vi "Main.vi"() -> ()   [LabVIEW 2020]
doc: "This template is for the Queued Message Handler design pattern.\n\nThe Event Handling Loop generates messages based on user interface actions.\n\nThe Message Handling Loop processes messages generated by the Event Handling Loop, or by other messages. The messages are string values, so new messages can be added easily to the Message Cases case structure in the Message Handling Loop. Each message cluster can also provide an optional value for Message Data, which is a variant that can be converted to whatever message-specific data is required."
uses:
  controls/UI Data.ctl
  support/Message Queue/Message Cluster.ctl
  <extravilib>/ChannelInstances/Messenger-t'Message Queue.lvlib-Message Cluster.ctl'/Write With Abort.vi
  <extravilib>/ChannelInstances/Messenger-t'Message Queue.lvlib-Message Cluster.ctl'/Instantiate.vi
  <extravilib>/ChannelInstances/Messenger-t'Message Queue.lvlib-Message Cluster.ctl'/Endpoint.vi
  <extravilib>/ChannelInstances/Event Messenger-bool/Instantiate.vi
  <extravilib>/ChannelInstances/Event Messenger-bool/))Channel.vi
  <vilib>/Utility/error.llb/Error Cluster From Error Code.vi
  <vilib>/ErrorRing/Error Ring.xnode
  <extravilib>/ChannelInstances/Event Messenger-bool.lvlib
  support/Message Queue/Message Queue.lvlib
  <extravilib>/ChannelInstances/Messenger-t'Message Queue.lvlib-Message Cluster.ctl'.lvlib
panel:
  in  "Button sin":bool
  in  "Button ^":bool
  in  "Button )":bool
  in  "Button (":bool
  in  "Button Ans":bool
  in  "Button E":bool
  in  "Button /":bool
  in  "Button *":bool
  in  "Button const pi":bool
  in  "Button -":bool
  in  "Button const e":bool
  in  "Button +":bool
  in  "Button Clear":bool
  in  "Button Del":bool
  in  "Button =":bool
  in  "Button .":bool
  in  "Button 9":bool
  in  "Button 8":bool
  in  "Button 7":bool
  in  "Button 6":bool
  in  "Button 5":bool
  in  "Button 4":bool
  in  "Button 3":bool
  in  "Button 2":bool
  in  "Button 1":bool
  out "Display":string
  in  "Button 0":bool
  in  "Exit":bool
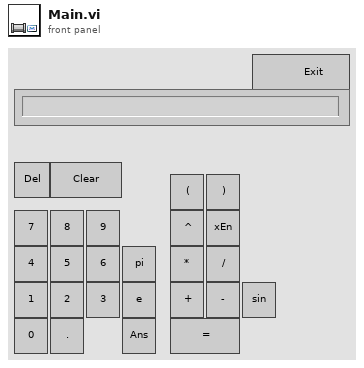
[diagram p1: front panel]
types:
  T1 = typedef "Message Queue.lvlib/Message Cluster.ctl" = cluster{"Message":string, "Message Data":variant}
  T2 = typedef "UI Data.ctl" = cluster{"Buttons to proces":string[], "Answer on display":bool, "Element type":string[], "Answer valid":bool, "Answer":string}
  T3 = typedef "Messenger-t'Message Queue.lvlib-Message Cluster.ctl'.lvlib/))Channel.ctl" = refnum<queue>
  T4 = cluster{"Strings to proces":string[], "Element type":string[]}
  T5 = cluster{"Buttons to proces":string[], "Element type":string[]}
  T6 = typedef "Event Messenger-bool.lvlib/))Channel.ctl" = refnum<queue>
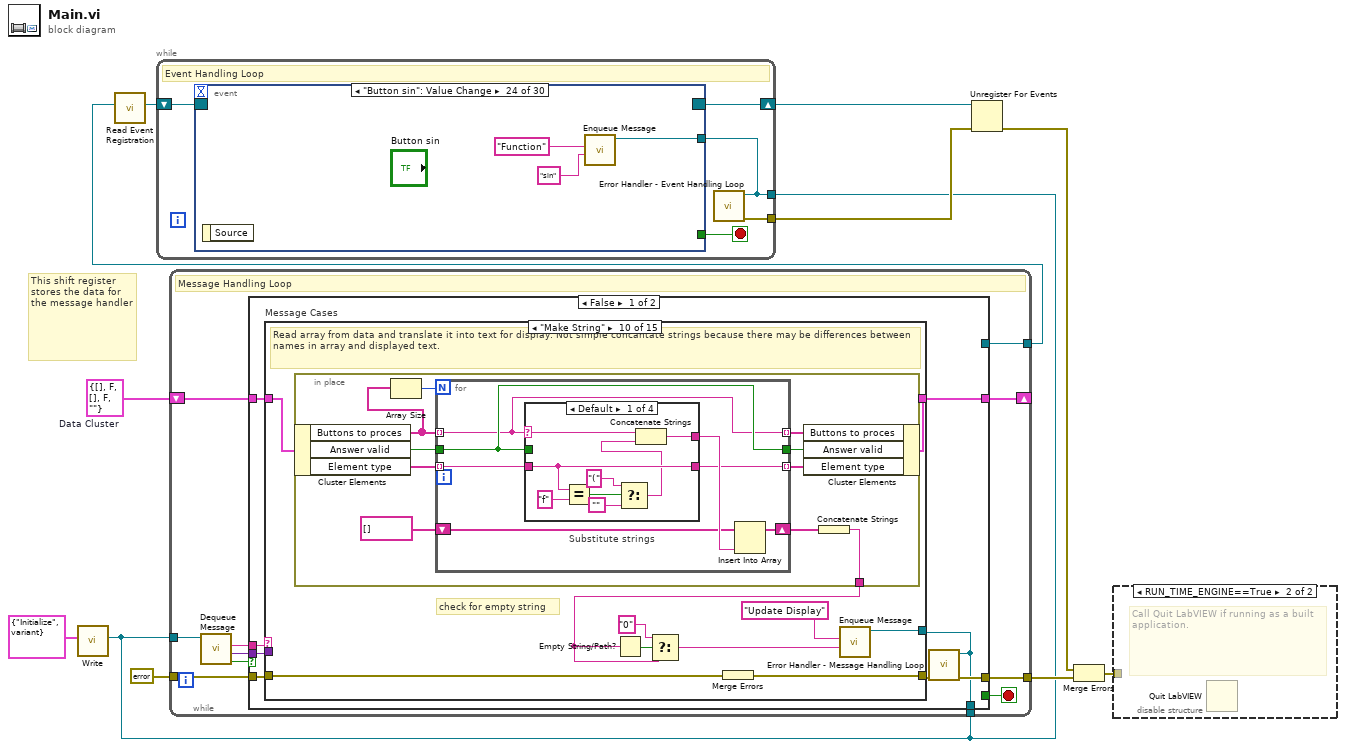
[diagram p0: block diagram]
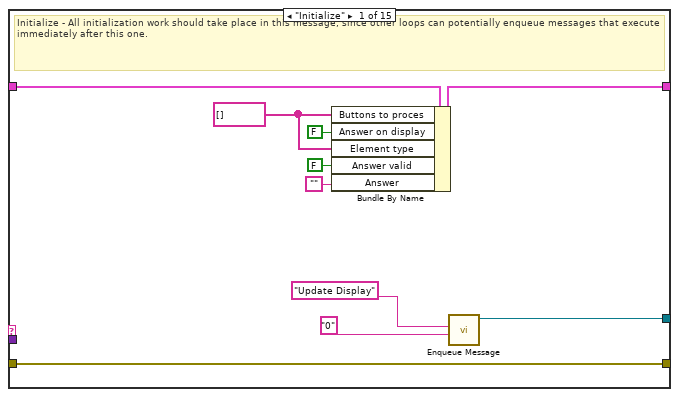
[diagram p2: hidden frame]
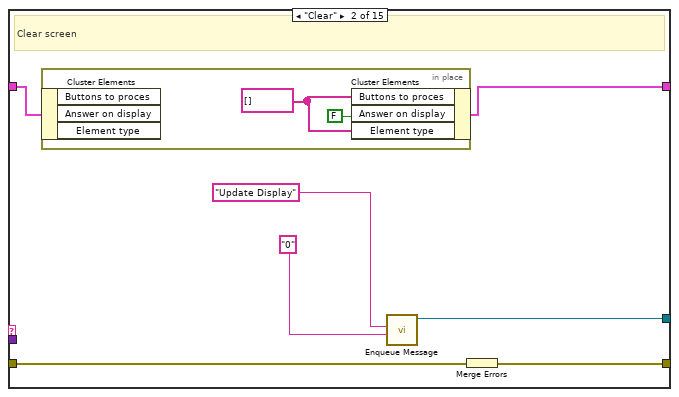
[diagram p3: hidden frame]
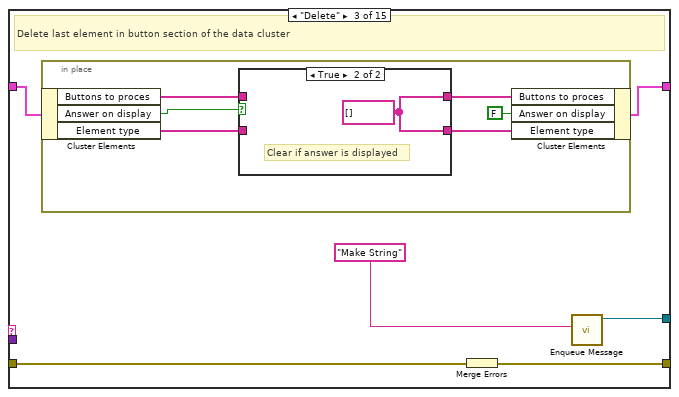
[diagram p4: hidden frame]
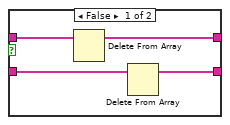
[diagram p5: hidden frame]
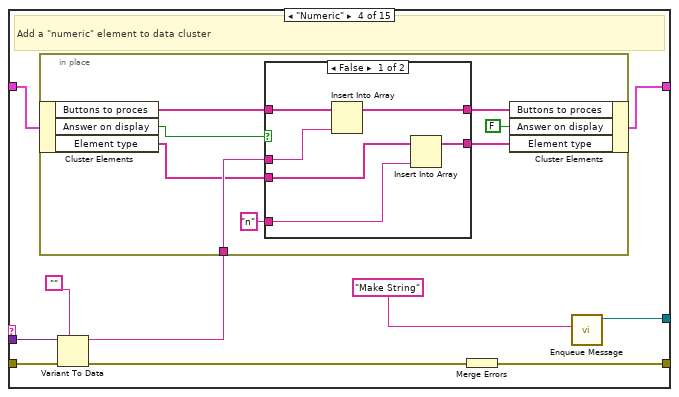
[diagram p6: hidden frame]
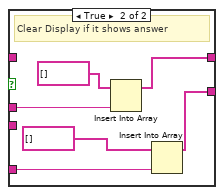
[diagram p7: hidden frame]
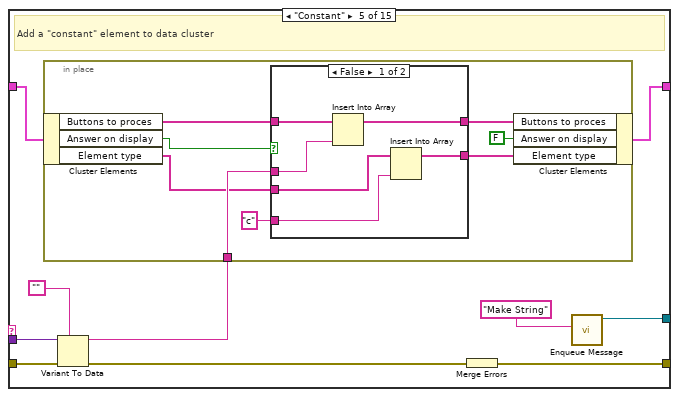
[diagram p8: hidden frame]
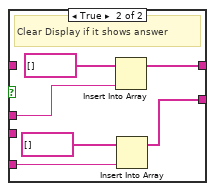
[diagram p9: hidden frame]
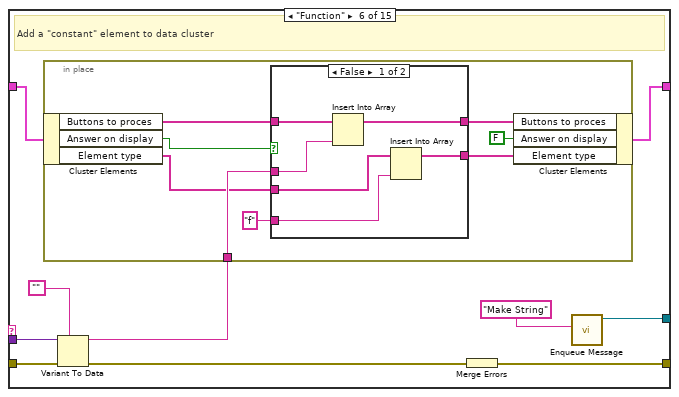
[diagram p10: hidden frame]
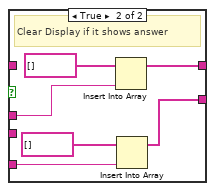
[diagram p11: hidden frame]
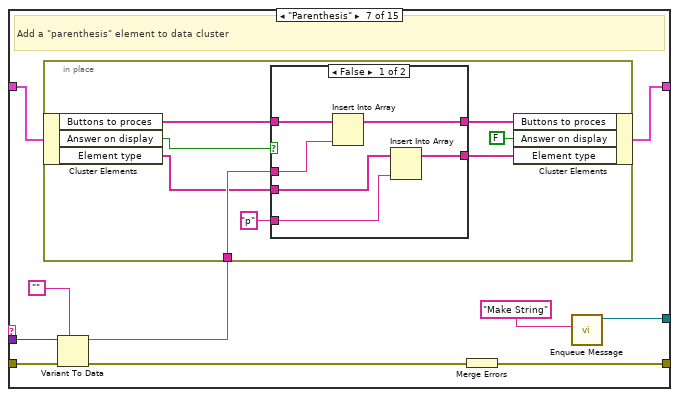
[diagram p12: hidden frame]
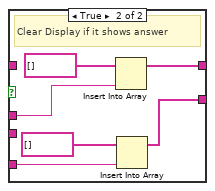
[diagram p13: hidden frame]
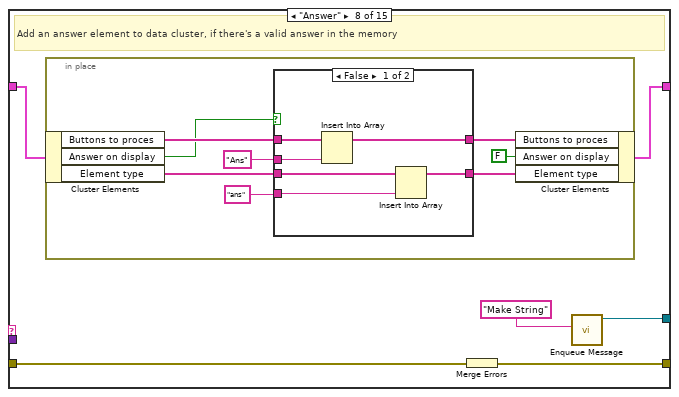
[diagram p14: hidden frame]
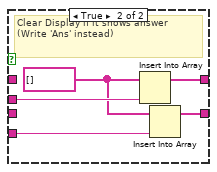
[diagram p15: hidden frame]
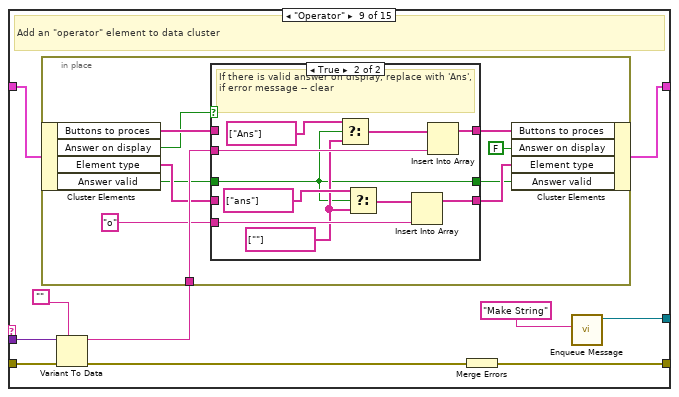
[diagram p16: hidden frame]
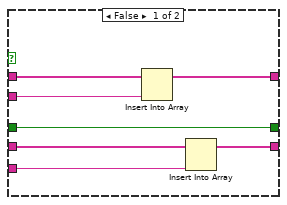
[diagram p17: hidden frame]
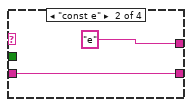
[diagram p18: hidden frame]
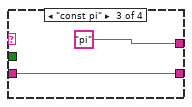
[diagram p19: hidden frame]
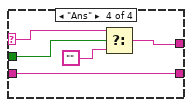
[diagram p20: hidden frame]
diagram:
  w8 = T2 {"Buttons to proces"=[], "Answer on display"=FALSE, "Element type"=[], "Answer valid"=FALSE, "Answer"=""}  # Data Cluster
  # "This shift register stores the data for the message handler"
  n1 = call <extravilib>:"Write.vi"("element"=T1 {"Message"="Initialize", "Message Data"=variant}) -> ("channel"=w2:T3)  [unwired: 8 in, 2 out]
  n2 = while {
    shift-right: [w21] -> _
    shift-left: w8 -> [w22]
    tunnel: [w19] -> w11
    tunnel: [w18] -> w6
    tunnel: w2 -> [w15]
    tunnel: errorcluster {"status"=FALSE, "code"=0, "source"=""} ("error IO") -> [w17]
    tunnel: w2 -> [w16]
    stop <- w20 stop-if-true
    # "Message Handling Loop"
    n3 = call "Dequeue Message.vi"("channel"=w15) -> ("channel aborted"=w12:bool, "message data"=w13:variant, "message"=w14:string)  [unwired: 8 in]
    n4 = case shown="False" w12 {
      tunnel: w22 -> [w30 w354]
      tunnel: [w29 w354] -> w21
      tunnel: [_ TRUE] -> w20
      tunnel: [w28 w355] -> w19
      tunnel: [_ w349] -> w18
      tunnel: w14 -> [w26 _]
      tunnel: w13 -> [w25 w351]
      tunnel: w17 -> [w24 w355]
      tunnel: [w23 _] -> w16
      frame False {
        n5 = case "Message Cases" shown="\"Make String\"" w26 {
          selector: w26 -> [_ _ _ _ _ _ _ _ _ _ _ _ _ _ w338]
          tunnel: w24 -> [w38 w46 w54 w69 w98 w128 w158 w191 w213 w257 w301 w325 w334 w337 _]
          tunnel: [w38 w47 w55 w76 w106 w136 w166 w192 w221 w258 w308 w326 w328 w335 w339] -> w27
          tunnel: w30 -> [w40 w42 w51 w73 w103 w133 w163 w188 w218 w254 w300 w327 w333 w336 w340]
          tunnel: [w39 w41 w50 w67 w102 w132 w162 w187 w214 w253 w303 w327 w333 w336 w340] -> w29
          tunnel: w25 -> [_ _ _ w72 w101 w131 w161 _ w217 _ _ w324 w332 _ _]
          tunnel: [w37 w45 w53 w75 w105 w135 w165 w190 w220 w256 w307 _ _ _ _] -> w23
          frame "Initialize" {
            w33 = string[] [] ("Buttons to proces")
            # "Initialize - All initialization work should take place in this message, since other loops can potentially enqueue messages that execute immediately after this one."
            n6 = Bundle By Name(cluster=w40, "Buttons to proces"=w33, "Answer on display"=FALSE, "Element type"=w33, "Answer valid"=FALSE, "Answer"="") -> (w39:T2)
            n7 = call "Enqueue Message.vi"("data (empty)"="0" ("Initial Message"), "message"="Update Display" ("Message")) -> ("channel"=w37:T3)  [unwired: 9 in]
          }
          frame "Clear" {
            # "Clear screen"
            n8 = in-place {
              w48 = string[] [] ("Buttons to proces")
              n9 = in-place-cluster #1(w42) -> ()  [unwired: 3 out]
              n10 = in-place-cluster #1("Buttons to proces"=w48, "Answer on display"=FALSE, "Element type"=w48) -> (w41:T2)
            }
            n11 = call "Enqueue Message.vi"("data (empty)"="0" ("\"Do Something\" button pressed"), "message"="Update Display" ("Message")) -> ("channel"=w45:T3)  [unwired: 9 in]
            n12 = Merge Errors(w46) -> (w47:errorcluster)
          }
          frame "Delete" {
            # "Delete last element in button section of the data cluster"
            n13 = in-place {
              n14 = in-place-cluster #2(w51) -> ("Buttons to proces"=w61:string[], "Answer on display"=w59:bool, "Element type"=w57:string[])
              n15 = case shown="True" w59 {
                tunnel: w61 -> [w65 _]
                tunnel: [w64 w66] -> w60
                tunnel: w57 -> [w63 _]
                tunnel: [w62 w66] -> w56
                frame False {
                  n16 = Delete From Array(array=w65) -> (array with subset deleted=w64:string[])  [unwired: 2 in, 1 out]
                  n17 = Delete From Array(array=w63) -> (array with subset deleted=w62:string[])  [unwired: 2 in, 1 out]
                }
                frame True {
                  w66 = string[] [] ("Buttons to proces")
                  # "Clear if answer is displayed"
                }
              }
              n18 = in-place-cluster #2("Buttons to proces"=w60, "Answer on display"=FALSE, "Element type"=w56) -> (w50:T2)
            }
            n19 = Merge Errors(w54) -> (w55:errorcluster)
            n20 = call "Enqueue Message.vi"("message"="Make String" ("Message")) -> ("channel"=w53:T3)  [unwired: 10 in]
          }
          frame "Numeric" {
            # "Add a \"numeric\" element to data cluster"
            n21 = Variant To Data(error in=w69, type="", Variant=w72) -> (data=w70:string, error out=w68:errorcluster)
            n22 = in-place {
              in-place-border: w70 -> [w84]
              n23 = in-place-cluster #3(w73) -> ("Buttons to proces"=w83:string[], "Answer on display"=w81:bool, "Element type"=w79:string[])
              n24 = case shown="False" w81 {
                tunnel: w84 -> [w90 w92]
                tunnel: w83 -> [w89 _]
                tunnel: [w88 w96] -> w82
                tunnel: w79 -> [w86 _]
                tunnel: [w87 w93] -> w78
                tunnel: "n" ("new element/subarray") -> [w85 w91]
                frame False {
                  n25 = Insert Into Array(array=w89, new element=w90) -> (w88:string[])  [unwired: 1 in]
                  n26 = Insert Into Array(array=w86, new element=w85) -> (w87:string[])  [unwired: 1 in]
                }
                frame True {
                  # "Clear Display if it shows answer"
                  n27 = Insert Into Array(array=string[] [] ("Buttons to proces"), new element=w92) -> (w96:string[])  [unwired: 1 in]
                  n28 = Insert Into Array(array=string[] [] ("Buttons to proces"), new element=w91) -> (w93:string[])  [unwired: 1 in]
                }
              }
              n29 = in-place-cluster #3("Buttons to proces"=w82, "Answer on display"=FALSE, "Element type"=w78) -> (w67:T2)
            }
            n30 = Merge Errors(w68) -> (w76:errorcluster)
            n31 = call "Enqueue Message.vi"("message"="Make String" ("Message")) -> ("channel"=w75:T3)  [unwired: 10 in]
          }
          frame "Constant" {
            # "Add a \"constant\" element to data cluster"
            n32 = Variant To Data(error in=w98, type="", Variant=w101) -> (data=w99:string, error out=w97:errorcluster)
            n33 = in-place {
              in-place-border: w99 -> [w114]
              n34 = in-place-cluster #4(w103) -> ("Buttons to proces"=w113:string[], "Answer on display"=w111:bool, "Element type"=w109:string[])
              n35 = case shown="False" w111 {
                tunnel: w114 -> [w120 w124]
                tunnel: w113 -> [w119 _]
                tunnel: [w118 w126] -> w112
                tunnel: w109 -> [w116 _]
                tunnel: [w117 w122] -> w108
                tunnel: "c" ("new element/subarray") -> [w115 w121]
                frame False {
                  n36 = Insert Into Array(array=w119, new element=w120) -> (w118:string[])  [unwired: 1 in]
                  n37 = Insert Into Array(array=w116, new element=w115) -> (w117:string[])  [unwired: 1 in]
                }
                frame True {
                  # "Clear Display if it shows answer"
                  n38 = Insert Into Array(array=string[] [] ("Buttons to proces"), new element=w124) -> (w126:string[])  [unwired: 1 in]
                  n39 = Insert Into Array(array=string[] [] ("Buttons to proces"), new element=w121) -> (w122:string[])  [unwired: 1 in]
                }
              }
              n40 = in-place-cluster #4("Buttons to proces"=w112, "Answer on display"=FALSE, "Element type"=w108) -> (w102:T2)
            }
            n41 = Merge Errors(w97) -> (w106:errorcluster)
            n42 = call "Enqueue Message.vi"("message"="Make String" ("Message")) -> ("channel"=w105:T3)  [unwired: 10 in]
          }
          frame "Function" {
            # "Add a \"constant\" element to data cluster"
            n43 = Variant To Data(error in=w128, type="", Variant=w131) -> (data=w129:string, error out=w127:errorcluster)
            n44 = in-place {
              in-place-border: w129 -> [w144]
              n45 = in-place-cluster #5(w133) -> ("Buttons to proces"=w143:string[], "Answer on display"=w141:bool, "Element type"=w139:string[])
              n46 = case shown="False" w141 {
                tunnel: w144 -> [w150 w154]
                tunnel: w143 -> [w149 _]
                tunnel: [w148 w156] -> w142
                tunnel: w139 -> [w146 _]
                tunnel: [w147 w152] -> w138
                tunnel: "f" ("new element/subarray") -> [w145 w151]
                frame False {
                  n47 = Insert Into Array(array=w149, new element=w150) -> (w148:string[])  [unwired: 1 in]
                  n48 = Insert Into Array(array=w146, new element=w145) -> (w147:string[])  [unwired: 1 in]
                }
                frame True {
                  # "Clear Display if it shows answer"
                  n49 = Insert Into Array(array=string[] [] ("Buttons to proces"), new element=w154) -> (w156:string[])  [unwired: 1 in]
                  n50 = Insert Into Array(array=string[] [] ("Buttons to proces"), new element=w151) -> (w152:string[])  [unwired: 1 in]
                }
              }
              n51 = in-place-cluster #5("Buttons to proces"=w142, "Answer on display"=FALSE, "Element type"=w138) -> (w132:T2)
            }
            n52 = Merge Errors(w127) -> (w136:errorcluster)
            n53 = call "Enqueue Message.vi"("message"="Make String" ("Message")) -> ("channel"=w135:T3)  [unwired: 10 in]
          }
          frame "Parenthesis" {
            # "Add a \"parenthesis\" element to data cluster"
            n54 = Variant To Data(error in=w158, type="", Variant=w161) -> (data=w159:string, error out=w157:errorcluster)
            n55 = in-place {
              in-place-border: w159 -> [w174]
              n56 = in-place-cluster #6(w163) -> ("Buttons to proces"=w173:string[], "Answer on display"=w171:bool, "Element type"=w169:string[])
              n57 = case shown="False" w171 {
                tunnel: w174 -> [w180 w184]
                tunnel: w173 -> [w179 _]
                tunnel: [w178 w186] -> w172
                tunnel: w169 -> [w176 _]
                tunnel: [w177 w182] -> w168
                tunnel: "p" ("new element/subarray") -> [w175 w181]
                frame False {
                  n58 = Insert Into Array(array=w179, new element=w180) -> (w178:string[])  [unwired: 1 in]
                  n59 = Insert Into Array(array=w176, new element=w175) -> (w177:string[])  [unwired: 1 in]
                }
                frame True {
                  # "Clear Display if it shows answer"
                  n60 = Insert Into Array(array=string[] [] ("Buttons to proces"), new element=w184) -> (w186:string[])  [unwired: 1 in]
                  n61 = Insert Into Array(array=string[] [] ("Buttons to proces"), new element=w181) -> (w182:string[])  [unwired: 1 in]
                }
              }
              n62 = in-place-cluster #6("Buttons to proces"=w172, "Answer on display"=FALSE, "Element type"=w168) -> (w162:T2)
            }
            n63 = Merge Errors(w157) -> (w166:errorcluster)
            n64 = call "Enqueue Message.vi"("message"="Make String" ("Message")) -> ("channel"=w165:T3)  [unwired: 10 in]
          }
          frame "Answer" {
            # "Add an answer element to data cluster, if there's a valid answer in the memory"
            n65 = in-place {
              n66 = in-place-cluster #7(w188) -> ("Buttons to proces"=w200:string[], "Answer on display"=w198:bool, "Element type"=w196:string[])
              n67 = case shown="False" w198 {
                tunnel: "Ans" -> [w206 w210]
                tunnel: w200 -> [w205 _]
                tunnel: [w204 w211] -> w199
                tunnel: w196 -> [w202 _]
                tunnel: [w203 w209] -> w195
                tunnel: "ans" -> [w201 w208]
                frame False {
                  n68 = Insert Into Array(array=w205, new element=w206) -> (w204:string[])  [unwired: 1 in]
                  n69 = Insert Into Array(array=w202, new element=w201) -> (w203:string[])  [unwired: 1 in]
                }
                frame True {
                  w207 = string[] [] ("Buttons to proces")
                  # "Clear Display if it shows answer \n(Write 'Ans' instead)"
                  n70 = Insert Into Array(array=w207, new element=w210) -> (w211:string[])  [unwired: 1 in]
                  n71 = Insert Into Array(array=w207, new element=w208) -> (w209:string[])  [unwired: 1 in]
                }
              }
              n72 = in-place-cluster #7("Buttons to proces"=w199, "Answer on display"=FALSE, "Element type"=w195) -> (w187:T2)
            }
            n73 = Merge Errors(w191) -> (w192:errorcluster)
            n74 = call "Enqueue Message.vi"("message"="Make String" ("Message")) -> ("channel"=w190:T3)  [unwired: 10 in]
          }
          frame "Operator" {
            # "Add an \"operator\" element to data cluster"
            n75 = Variant To Data(error in=w213, type="", Variant=w217) -> (data=w215:string, error out=w212:errorcluster)
            n76 = in-place {
              in-place-border: w215 -> [w231]
              n77 = in-place-cluster #8(w218) -> ("Buttons to proces"=w230:string[], "Answer on display"=w229:bool, "Element type"=w227:string[], "Answer valid"=w223:bool)
              n78 = case shown="True" w229 {
                tunnel: w231 -> [w238 w247]
                tunnel: w230 -> [w237 _]
                tunnel: [w236 w248] -> w224
                tunnel: w227 -> [w234 _]
                tunnel: [w235 w246] -> w225
                tunnel: "o" ("new element/subarray") -> [w233 w245]
                tunnel: w223 -> [w232 w239]
                tunnel: [w232 w239] -> w222
                frame False {
                  n79 = Insert Into Array(array=w237, new element=w238) -> (w236:string[])  [unwired: 1 in]
                  n80 = Insert Into Array(array=w234, new element=w233) -> (w235:string[])  [unwired: 1 in]
                }
                frame True {
                  w240 = string[] [""] ("Buttons to proces")
                  # "If there is valid answer on display, replace with 'Ans', if error message -- clear"
                  n81 = Select(t=string[] ["Ans"] ("Buttons to proces"), s=w239, f=w240) -> (s? t:f=w244:string[])
                  n82 = Select(t=string[] ["ans"] ("Buttons to proces"), s=w239, f=w240) -> (s? t:f=w243:string[])
                  n83 = Insert Into Array(array=w243, new element=w245) -> (w246:string[])  [unwired: 1 in]
                  n84 = Insert Into Array(array=w244, new element=w247) -> (w248:string[])  [unwired: 1 in]
                }
              }
              n85 = in-place-cluster #8("Buttons to proces"=w224, "Answer on display"=FALSE, "Element type"=w225, "Answer valid"=w222) -> (w214:T2)
            }
            n86 = Merge Errors(w212) -> (w221:errorcluster)
            n87 = call "Enqueue Message.vi"("message"="Make String" ("Message")) -> ("channel"=w220:T3)  [unwired: 10 in]
          }
          frame "Make String" {
            # "check for empty string"
            # "Read array from data and translate it into text for display. Not simple concantate strings because there may be differences between names in array and displayed text."
            n88 = in-place {
              in-place-border: [w265] -> w250
              n89 = in-place-cluster #9(w254) -> ("Buttons to proces"=w259:string[], "Answer valid"=w262:bool, "Element type"=w261:string[])
              n90 = Array Size(array=w259) -> (size(s)=w267:i32)
              n91 = for {
                N: w267 -> [_]
                tunnel: [w269] -> w268 mode=indexing
                shift-right: [w275] -> w266
                shift-left: string[] [] ("Buttons to proces") -> [w271]
                tunnel: [w270] -> w263
                tunnel: w262 -> [w270]
                tunnel: w261 -> [w272] mode=indexing
                tunnel: w259 -> [w269] mode=indexing
                tunnel: [w273] -> w260 mode=indexing
                n92 = case "Substitute strings" shown="Default" w269 {
                  selector: w269 -> [w283 _ _ w290]
                  tunnel: w270 -> [_ _ _ w292]
                  tunnel: [w280 "e" "pi" w289] -> w274
                  tunnel: [w282 w284 w286 w288] -> w273
                  tunnel: w272 -> [w282 w284 w286 w288]
                  frame Default {
                    n93 = Equal?(x=w282, y="f") -> (x = y?=w279:bool)
                    n94 = Select(t="(", s=w279, f="") -> (s? t:f=w276:string)
                    n95 = Concatenate Strings(w283, w276) -> (w280:string)
                  }
                  frame "const e" {
                  }
                  frame "const pi" {
                  }
                  frame "Ans" {
                    n96 = Select(t=w290, s=w292, f="") -> (s? t:f=w289:string)
                  }
                }
                n97 = Insert Into Array(array=w271, new element=w274) -> (w275:string[])  [unwired: 1 in]
              }
              n98 = in-place-cluster #9("Buttons to proces"=w268, "Answer valid"=w263, "Element type"=w260) -> (w253:T2)
              n99 = Concatenate Strings(w266) -> (w265:string)
            }
            n100 = Empty String/Path?(string/path=w250) -> (empty?=w252:bool)
            n101 = Select(t="0" ("\"Do Something\" button pressed"), s=w252, f=w250) -> (s? t:f=w249:string)
            n102 = Merge Errors(w257) -> (w258:errorcluster)
            n103 = call "Enqueue Message.vi"("data (empty)"=w249, "message"="Update Display" ("Message")) -> ("channel"=w256:T3)  [unwired: 9 in]
          }
          frame "Execute" {
            w296 = i32[] [100004, 100005, 100007, 100008, 100009]  # ignored errors
            # "Run solver. (At present in three parts. Prepare table. Convert to postfix notation. Solve.)\nShow answer (or solver error message) on display.\nIf answer is valid, write it into memory."
            n104 = call "data preparer.vi"("error in (no error)"=w301, "UI Data"=w300) -> ("error out"=w304:errorcluster, "Prepared (Infix) Data"=w305:T4)
            n105 = call "Shunting yard algorithm.vi"("error in (no error)"=w304, "Infix Notation Data"=w305) -> ("error out"=w298:errorcluster, "Postfix Notation Data"=w302:T5)
            n106 = call "RPN Arithmetic Solver.vi"("Solver Input (Postfix) Data"=w302, "error in (no error)"=w298) -> ("Answer (string)"=w299:string, "error out"=w295:errorcluster)  [unwired: 1 in, 1 out]
            n107 = Unbundle By Name(w295) -> ("status"=w294:bool)
            n108 = call "Ignore error from the list.vi"("error codes to ignore"=w296, "error in (no error)"=w295) -> ("error out"=w297:errorcluster)
            n109 = Not(x=w294) -> (.not. x?=w293:bool)
            n110 = case shown="True" w293 {
              tunnel: [w310 w314] -> w303
              tunnel: w299 -> [_ w315]
              tunnel: w300 -> [w309 w320]
              frame False {
                n111 = Bundle By Name(cluster=w309, "Buttons to proces"=string[] [], "Answer on display"=TRUE, "Element type"=string[] [""] ("Buttons to proces")) -> (w310:T2)
              }
              frame True {
                n112 = Bundle By Name(cluster=w320, "Buttons to proces"=string[] ["Ans"], "Answer on display"=TRUE ("Answer valid"), "Element type"=string[] ["ans"], "Answer valid"=TRUE ("Answer on display"), "Answer"=w315) -> (w314:T2)
              }
            }
            n113 = Merge Errors(w297) -> (w308:errorcluster)
            n114 = call "Enqueue Message.vi"("data (empty)"=w299, "message"="Update Display" ("Message")) -> ("channel"=w307:T3)  [unwired: 9 in]
          }
          frame "Update Display" {
            # "#CodeRecommended - If you wish to decouple the Message Handling Loop from your user interface, consider creating User Events (like the \"Stop\" event in this VI) to message the Event Handling Loop whenever the user interface needs updating."
            # "Update Display - Convert the message data to a string to display in the Data Display indicator."
            n115 = Variant To Data(error in=w325, type="", Variant=w324) -> (data=→"Display":string, error out=w322:errorcluster)
            n116 = Merge Errors(w322) -> (w326:errorcluster)
          }
          frame "Error" {
            # "#CodeRecommended - If you ever change the name of this \"Error\" message, you'll need to update the name in the Check Loop Error.vi as well."
            # "#CodeRecommended - Consider creating a system for logging errors in some way. These errors are for notification purposes only. Handling of specific errors should be performed in the message frames that generated the error."
            # "Error - Display an error dialog. This message is sent by the \"Error Handler\" VIs at the end of other loops in this application."
            n117 = Variant To Data(error in=w334, type=errorcluster {"status"=FALSE, "code"=0, "source"=""} ("error constant"), Variant=w332) -> (data=w330:errorcluster, error out=w329:errorcluster)
            n118 = call <vilib>:"Simple Error Handler.vi"("error in (no error)"=w330) -> ()  [unwired: 4 in, 5 out]
            n119 = Merge Errors(w329) -> (w328:errorcluster)
          }
          frame "---Copy This Frame---" {
            # "Duplicate this frame when creating new messages.  Change this comment in the duplicated frame to describe this message."
            n120 = Merge Errors(w337) -> (w335:errorcluster)
          }
          frame Default {
            # "'Default' case only runs if there is a message that isn't defined in any of the other cases.  Output a programming error."
            n121 = xnode "Error Ring"("parameter 0"=w338) -> ("error out"=w339:errorcluster)
          }
        }
        n122 = call "Error Handler - Message Handling Loop.vi"("channel"=w23, "error in (no error)"=w27) -> ("dup error in"=w28:errorcluster)  [unwired: 9 in]
      }
      frame True {
        w350 = TRUE  # Exit
        # "Tell the event loop to stop if it has not done so already."
        # "Ignore error out here. If the Exit message was sent without an attached error, that is fine."
        # "#CodeNeeded - Add any required cleanup code here, such as putting hardware into a safe mode. Note that if 'Exit' was called as a result of an error, an error dialog will be displayed. Add any custom error handling for an 'Exit' condition here as well."
        # "Shutdown routine."
        n123 = Variant To Data(type=errorcluster {"status"=FALSE, "code"=0, "source"=""} ("error constant"), Variant=w351) -> (data=w352:errorcluster)  [unwired: 1 in, 1 out]
        n124 = call <vilib>:"Simple Error Handler.vi"("error in (no error)"=w352) -> ()  [unwired: 4 in, 5 out]
        n125 = local write "Display"("" ("Exit Application")) -> ()
        n126 = call <extravilib>:"Write.vi"("element"=w350) -> ("channel"=w349:T6)  [unwired: 9 in, 1 out]
      }
    }
  }
  n127 = call <extravilib>:"Read Event Registration.vi"("channel"=w6) -> ("event registration refnum"=w5:refnum<event-registration>)  [unwired: 10 in]
  n128 = while {
    shift-right: [w360] -> w9
    shift-left: w5 -> [w361]
    tunnel: [w358] -> w7
    tunnel: w2 -> [w357]
    stop <- w359 stop-if-true
    # "Event Handling Loop"
    n129 = event shown="[23] \"Button sin\": Value Change" {
      selector: w361 -> [_ _ _ _ _ _ _ _ _ _ _ _ _ _ _ _ _ _ _ _ _ _ _ _ _ _ _ _ _ _]
      dyn-events: [_ _ _ _ _ _ _ _ _ _ _ _ _ _ _ _ _ _ _ _ _ _ _ _ _ _ _ _ _ _] -> w360
      timeout: _ -> [_ _ _ _ _ _ _ _ _ _ _ _ _ _ _ _ _ _ _ _ _ _ _ _ _ _ _ _ _ _]
      tunnel: [_ _ _ _ _ _ _ _ _ _ _ _ _ _ _ _ _ _ _ _ _ _ _ _ _ _ w436 _ w439 TRUE ("Discard?")] -> w359
      tunnel: [w364 w367 w368 w371 w374 w377 w380 w383 w386 w389 w392 w395 w398 w401 w404 w406 w409 w412 w415 w418 w421 w424 w427 w430 w432 w434 w437 _ w440 _] -> w357
      event "Button 0": Value Change {
        n130 = event-data() -> ()  [unwired: 1 in, 1 out]
        n131 = call "Enqueue Message.vi"("data (empty)"="0", "message"="Numeric" ("Message")) -> ("channel"=w364:T3)  [unwired: 9 in]
      }
      event "Button 1": Value Change {
        n132 = event-data() -> ()  [unwired: 1 in, 1 out]
        n133 = call "Enqueue Message.vi"("data (empty)"="1", "message"="Numeric" ("Message")) -> ("channel"=w367:T3)  [unwired: 9 in]
      }
      event "Button 2": Value Change {
        n134 = event-data() -> ()  [unwired: 1 in, 1 out]
        n135 = call "Enqueue Message.vi"("data (empty)"="2", "message"="Numeric" ("Message")) -> ("channel"=w368:T3)  [unwired: 9 in]
      }
      event "Button 3": Value Change {
        n136 = event-data() -> ()  [unwired: 1 in, 1 out]
        n137 = call "Enqueue Message.vi"("data (empty)"="3", "message"="Numeric" ("Message")) -> ("channel"=w371:T3)  [unwired: 9 in]
      }
      event "Button 4": Value Change {
        n138 = event-data() -> ()  [unwired: 1 in, 1 out]
        n139 = call "Enqueue Message.vi"("data (empty)"="4", "message"="Numeric" ("Message")) -> ("channel"=w374:T3)  [unwired: 9 in]
      }
      event "Button 5": Value Change {
        n140 = event-data() -> ()  [unwired: 1 in, 1 out]
        n141 = call "Enqueue Message.vi"("data (empty)"="5", "message"="Numeric" ("Message")) -> ("channel"=w377:T3)  [unwired: 9 in]
      }
      event "Button 6": Value Change {
        n142 = event-data() -> ()  [unwired: 1 in, 1 out]
        n143 = call "Enqueue Message.vi"("data (empty)"="6", "message"="Numeric" ("Message")) -> ("channel"=w380:T3)  [unwired: 9 in]
      }
      event "Button 7": Value Change {
        n144 = event-data() -> ()  [unwired: 1 in, 1 out]
        n145 = call "Enqueue Message.vi"("data (empty)"="7", "message"="Numeric" ("Message")) -> ("channel"=w383:T3)  [unwired: 9 in]
      }
      event "Button 8": Value Change {
        n146 = event-data() -> ()  [unwired: 1 in, 1 out]
        n147 = call "Enqueue Message.vi"("data (empty)"="8", "message"="Numeric" ("Message")) -> ("channel"=w386:T3)  [unwired: 9 in]
      }
      event "Button 9": Value Change {
        n148 = event-data() -> ()  [unwired: 1 in, 1 out]
        n149 = call "Enqueue Message.vi"("data (empty)"="9", "message"="Numeric" ("Message")) -> ("channel"=w389:T3)  [unwired: 9 in]
      }
      event "Button .": Value Change {
        n150 = event-data() -> ()  [unwired: 1 in, 1 out]
        n151 = call "Enqueue Message.vi"("data (empty)"=".", "message"="Numeric" ("Message")) -> ("channel"=w392:T3)  [unwired: 9 in]
      }
      event "Button E": Value Change {
        n152 = event-data() -> ()  [unwired: 1 in, 1 out]
        n153 = call "Enqueue Message.vi"("data (empty)"="E", "message"="Operator" ("Message")) -> ("channel"=w395:T3)  [unwired: 9 in]
      }
      event "Button const e": Value Change {
        n154 = event-data() -> ()  [unwired: 1 in, 1 out]
        n155 = call "Enqueue Message.vi"("data (empty)"="const e", "message"="Constant" ("Message")) -> ("channel"=w398:T3)  [unwired: 9 in]
      }
      event "Button const pi": Value Change {
        n156 = event-data() -> ()  [unwired: 1 in, 1 out]
        n157 = call "Enqueue Message.vi"("data (empty)"="const pi", "message"="Constant" ("Message")) -> ("channel"=w401:T3)  [unwired: 9 in]
      }
      event "Button Ans": Value Change {
        n158 = event-data() -> ()  [unwired: 1 in, 1 out]
        n159 = call "Enqueue Message.vi"("message"="Answer" ("Message")) -> ("channel"=w404:T3)  [unwired: 10 in]
      }
      event "Button +": Value Change {
        n160 = event-data() -> ()  [unwired: 1 in, 1 out]
        n161 = call "Enqueue Message.vi"("data (empty)"="+", "message"="Operator" ("Message")) -> ("channel"=w406:T3)  [unwired: 9 in]
      }
      event "Button -": Value Change {
        n162 = event-data() -> ()  [unwired: 1 in, 1 out]
        n163 = call "Enqueue Message.vi"("data (empty)"="-", "message"="Operator" ("Message")) -> ("channel"=w409:T3)  [unwired: 9 in]
      }
      event "Button *": Value Change {
        n164 = event-data() -> ()  [unwired: 1 in, 1 out]
        n165 = call "Enqueue Message.vi"("data (empty)"="*", "message"="Operator" ("Message")) -> ("channel"=w412:T3)  [unwired: 9 in]
      }
      event "Button /": Value Change {
        n166 = event-data() -> ()  [unwired: 1 in, 1 out]
        n167 = call "Enqueue Message.vi"("data (empty)"="/", "message"="Operator" ("Message")) -> ("channel"=w415:T3)  [unwired: 9 in]
      }
      event "Button ^": Value Change {
        n168 = event-data() -> ()  [unwired: 1 in, 1 out]
        n169 = call "Enqueue Message.vi"("data (empty)"="^", "message"="Operator" ("Message")) -> ("channel"=w418:T3)  [unwired: 9 in]
      }
      event "Button =": Value Change {
        n170 = event-data() -> ()  [unwired: 1 in, 1 out]
        n171 = call "Enqueue Message.vi"("message"="Execute" ("Message")) -> ("channel"=w421:T3)  [unwired: 10 in]
      }
      event "Button (": Value Change {
        n172 = event-data() -> ()  [unwired: 1 in, 1 out]
        n173 = call "Enqueue Message.vi"("data (empty)"="(", "message"="Parenthesis" ("Message")) -> ("channel"=w424:T3)  [unwired: 9 in]
      }
      event "Button )": Value Change {
        n174 = event-data() -> ()  [unwired: 1 in, 1 out]
        n175 = call "Enqueue Message.vi"("data (empty)"=")", "message"="Parenthesis" ("Message")) -> ("channel"=w427:T3)  [unwired: 9 in]
      }
      event "Button sin": Value Change {
        n176 = event-data() -> ()  [unwired: 1 in, 1 out]
        n177 = call "Enqueue Message.vi"("data (empty)"="sin", "message"="Function" ("Message")) -> ("channel"=w430:T3)  [unwired: 9 in]
      }
      event "Button Del": Value Change {
        n178 = event-data() -> ()  [unwired: 1 in, 1 out]
        n179 = call "Enqueue Message.vi"("message"="Delete" ("Message")) -> ("channel"=w432:T3)  [unwired: 10 in]
      }
      event "Button Clear": Value Change {
        n180 = event-data() -> ()  [unwired: 1 in, 1 out]
        n181 = call "Enqueue Message.vi"("message"="Clear" ("Message")) -> ("channel"=w434:T3)  [unwired: 10 in]
      }
      event Panel Close? {
        # "Ask user to confirm quit, which will send the exit message if the user says yes. Regardless of the user's response, discard the event so the Exit message has a chance to run to clean up the application."
        n182 = event-data() -> ()  [unwired: 1 in, 1 out]
        n183 = call "Error Handler - Confirm Quit.vi"() -> ("exit confirmed"=w436:bool, "channel"=w437:T3)  [unwired: 10 in]
        n184 = event-data("Discard?"=TRUE) -> ()  [unwired: 1 in, 1 out]
      }
      event Application Instance Close {
        # "#CodeRecommended - When a project closes, all VIs within that project are aborted and leave memory. However, any code placed in this event frame is guaranteed to run to completion, so add any cleanup code that absolutely must happen here when working in the development environment. Normal shutdown code should go in the \"aborted=true\" frame in the Message Handling Loop."
        n185 = event-data() -> ()  [unwired: 1 in, 1 out]
      }
      event "Exit": Value Change {
        n186 = event-data() -> ()  [unwired: 1 in, 1 out]
        n187 = call "Error Handler - Confirm Quit.vi"() -> ("exit confirmed"=w439:bool, "channel"=w440:T3)  [unwired: 10 in]
      }
      event User Event {
        # "The Message Handling Loop processed an \"Exit\" message, which fired this event to stop the Event Handling Loop."
        n188 = event-data() -> ()  [unwired: 1 in, 1 out]
      }
    }
    n189 = call "Error Handler - Event Handling Loop.vi"("channel"=w357) -> ("dup error in"=w358:errorcluster)  [unwired: 10 in]
  }
  n190 = Unregister For Events(event registration refnum=w9, error in=w7) -> (error out=w10:errorcluster)
  n191 = Merge Errors(w10, w11) -> (w4:errorcluster)
  n192 = disable-structure shown="RUN_TIME_ENGINE==True" {
    disable-tunnel: w4 -> [_ _]
    frame condition #0 (active) {
    }
    frame condition #1 {
      # "Call Quit LabVIEW if running as a built application."
      n193 = Quit LabVIEW() -> ()  [unwired: 1 in]
    }
  }
